vi "Write DAQ Data.vi"(8 "error in (no error)":errorcluster, 9 "Voltage with Time":dbl[][](array[numeric]), 10 "File Infor":T1, 11 "CSV File in":refnum<class "CSV File.lvclass">) -> (0 "error out":errorcluster, 3 "CSV File out":refnum<class "CSV File.lvclass">)   [LabVIEW 2021, in "CSV File.lvclass"]
doc: "This vi helps to write Voltage with Time 2 dimensional array into CSV file."
uses:
  CSV File.lvclass
  Control/File Information Cluster.ctl
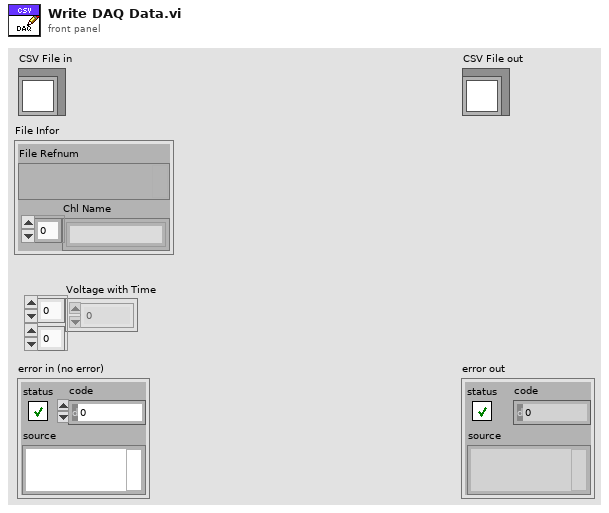
[diagram p1: front panel]
types:
  T1 = typedef "File Information Cluster.ctl" = cluster{"File Refnum":variant, "Chl Name":string[]}
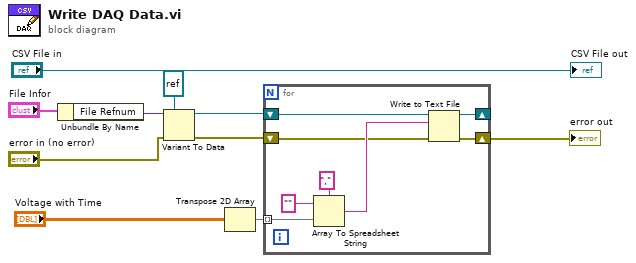
[diagram p0: block diagram]
diagram:
  n1 = Unbundle By Name("File Infor") -> ("File Refnum"=w3:variant)
  n2 = Variant To Data(error in="error in (no error)", type=refnum<file> refnum ("CSV Refnum"), Variant=w3) -> (data=w5:refnum<file>, error out=w6:errorcluster)
  n3 = Transpose 2D Array(2D array="Voltage with Time") -> (transposed array=w4:dbl[][])
  n4 = for {
    tunnel: w4 -> [w16] mode=indexing
    shift-right: [w13] -> _
    shift-left: w5 -> [w14]
    shift-right: [w12] -> w10
    shift-left: w6 -> [w11]
    n5 = Array To Spreadsheet String(delimiter (Tab)=",", array=w16, 3:"" ("format string")) -> (spreadsheet string=w15:string)
    n6 = Write to Text File(file (use dialog)=w14, text=w15, error in=w11) -> (refnum out=w13:refnum<file>, error out=w12:errorcluster)  [unwired: 1 in, 1 out]
  }
  "error out" <- w10
  "CSV File out" <- "CSV File in"
